vi "Create.vi"(8 "error in (no error)":errorcluster, 10 "Show Send?":bool) -> (0 "error out":errorcluster, 3 "Filter by Process out":refnum<class "Filter by Is Send.lvclass">)   [LabVIEW 2020, in "Filter by Is Send.lvclass"]
uses:
  Filter by Is Send.lvclass
  Filter by Is Send.lvclass/Filter by Is Send.ctl
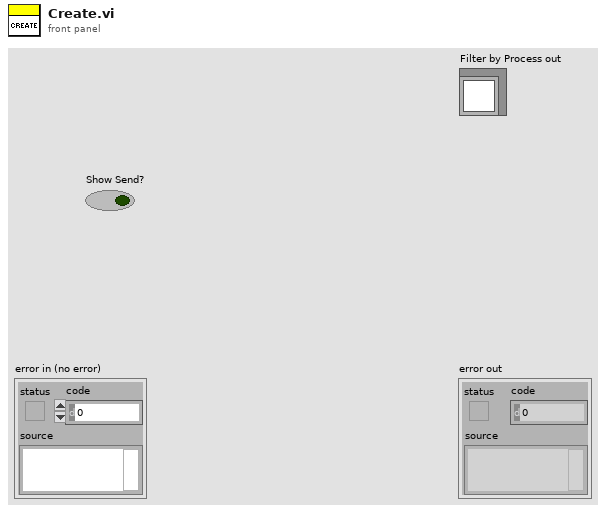
[diagram p1: front panel]
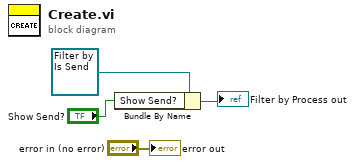
[diagram p0: block diagram]
diagram:
  n1 = Bundle By Name(cluster=refnum<class "Filter by Is Send.lvclass"> refnum ("Filter by Process out"), "Show Send?"="Show Send?") -> (→"Filter by Process out":refnum<class "Filter by Is Send.lvclass">)
  "error out" <- "error in (no error)"
